vi "DataHeader.vi"(8 "Script #":i32, 9 "Scripting":bool) -> (0 "error out":errorcluster, 2 "Timestamp":string, 3 "refnum out":refnum<file>)   [LabVIEW 2018]
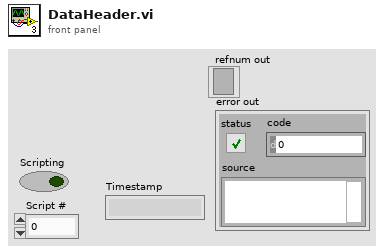
[diagram p1: front panel]
types:
  T1 = enum16{"open", "replace", "create", "open or create", "replace or create", "replace or create with confirmation"}
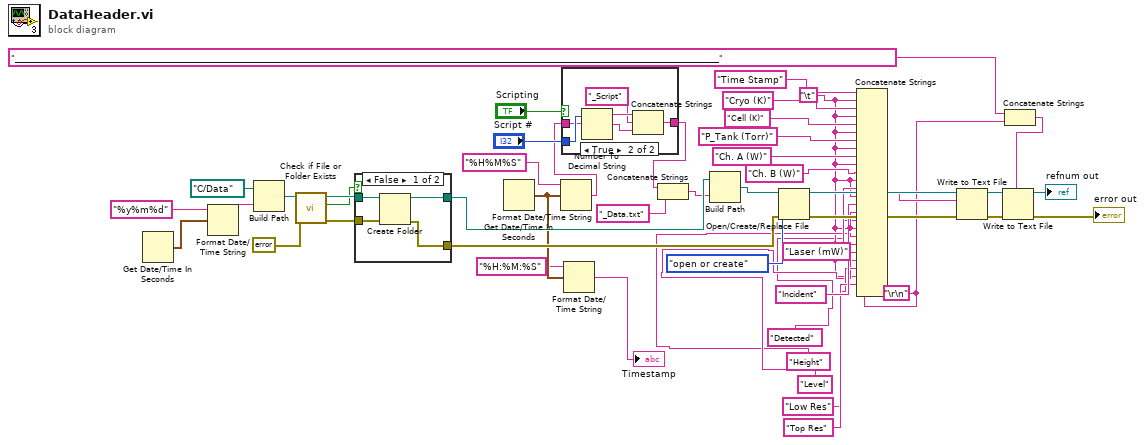
[diagram p0: block diagram]
diagram:
  w7 = "\r\n"
  w2 = "\t"
  n1 = Get Date/Time In Seconds() -> (seconds since 1Jan1904=w46:timestamp)
  n2 = Format Date/Time String(time format string (%c)="%y%m%d", seconds (now)=w46) -> (date/time string=w45:string)  [unwired: 1 in]
  n3 = Build Path(base path=path "C:/Data", name or relative path=w45) -> (appended path=w44:path)
  n4 = call <vilib>:"Check if File or Folder Exists.vi"("error in (no error)"=errorcluster {"status"=FALSE, "code"=0, "source"=""}, "path"=w44) -> ("error out"=w39:errorcluster, "file or folder exists?"=w42:bool, "dup path"=w43:path)  [unwired: 7 in]
  n5 = case shown="False" w42 {
    tunnel: w43 -> [w51 w53]
    tunnel: [w50 w53] -> w40
    tunnel: w39 -> [w49 w52]
    tunnel: [w48 w52] -> w37
    frame False {
      n6 = Create Folder(path (use dialog)=w51, error in=w49) -> (created path=w50:path, error out=w48:errorcluster)  [unwired: 1 in, 1 out]
    }
    frame True {
    }
  }
  n7 = Get Date/Time In Seconds() -> (seconds since 1Jan1904=w12:timestamp)
  n8 = Format Date/Time String(time format string (%c)="%H%M%S", seconds (now)=w12) -> (date/time string=w13:string)  [unwired: 1 in]
  n9 = case shown="True" "Scripting" {
    tunnel: "Script #" -> [_ w59]
    tunnel: w13 -> [w54 w57]
    tunnel: [w54 w58] -> w14
    frame False {
    }
    frame True {
      n10 = Number To Decimal String(number=w59) -> (decimal integer string=w56:string)  [unwired: 1 in]
      n11 = Concatenate Strings(w57, "_Script" ("string"), w56) -> (w58:string)
    }
  }
  n12 = Format Date/Time String(time format string (%c)="%H:%M:%S", seconds (now)=w12) -> (date/time string=→"Timestamp":string)  [unwired: 1 in]
  n13 = Concatenate Strings(w14, "_Data.txt" ("input 2")) -> (w15:string)
  n14 = Build Path(base path=w40, name or relative path=w15) -> (appended path=w38:path)
  n15 = Open/Create/Replace File(file path (use dialog)=w38, error in=w37, operation (0:open)=T1."open or create") -> (refnum out=w35:refnum<file>, error out=w36:errorcluster)  [unwired: 3 in, 1 out]
  n16 = Concatenate Strings("Time Stamp" ("string"), w2, "Cryo (K)" ("string"), w2, "Cell (K)" ("string"), w2, "P_Tank (Torr)" ("string"), w2, "Ch. A (W)" ("string"), w2, "Ch. B (W)" ("string"), w2, "Laser (mW)" ("string"), w2, "Incident" ("string"), w2, "Detected" ("string"), w2, "Height" ("string"), w2, "Level" ("string"), w2, "Low Res" ("string"), w2, "Top Res" ("string"), w7) -> (w28:string)
  n17 = Write to Text File(file (use dialog)=w35, text=w28, error in=w36) -> (refnum out=w33:refnum<file>, error out=w34:errorcluster)  [unwired: 1 in, 1 out]
  n18 = Concatenate Strings("________________________________________________________________________________________________________________________________________________________________________________" ("text"), w7) -> (w26:string)
  n19 = Write to Text File(file (use dialog)=w33, text=w26, error in=w34) -> (refnum out=→"refnum out":refnum<file>, error out=→"error out":errorcluster)  [unwired: 1 in, 1 out]
